vi "Read Sequence Element Configuration.vi"(8 "error in (no error)":errorcluster, 11 "Sequence Element in":refnum<class "Sequence Element.lvclass">) -> (0 "error out":errorcluster, 2 "Configuration":T1 {"Duration" format="%#_6ps"}, 3 "Sequence Element out":refnum<class "Sequence Element.lvclass">)   [LabVIEW 2016, in "Sequence Element.lvclass"]
uses:
  Sequence Element.lvclass
  C:/github/Measure_core/da Base/Template Module.lvclass
  Sequence Element Configuration.ctl
  Template Module/Template Module.lvclass/Template Module.ctl
  Template Module/Read Configuration.vi
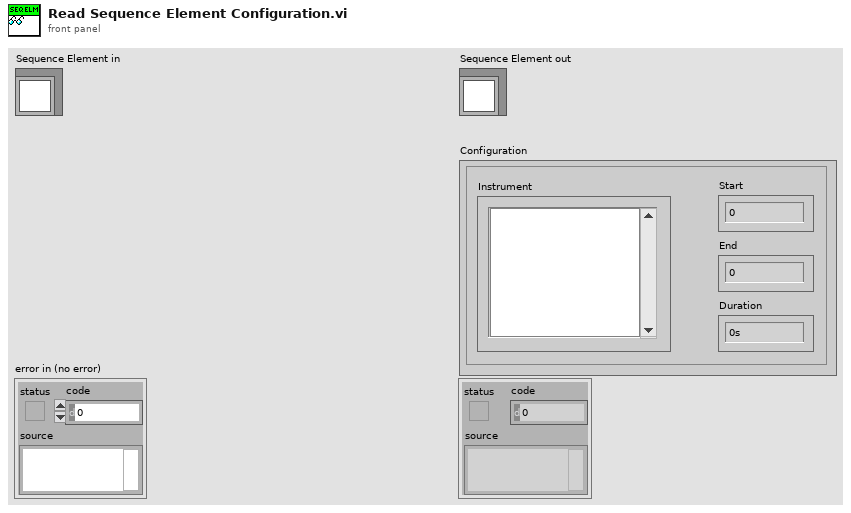
[diagram p1: front panel]
types:
  T1 = typedef "Sequence Element Configuration.ctl" = cluster{"Start":dbl, "End":dbl, "Duration":dbl, "Instrument":i32}
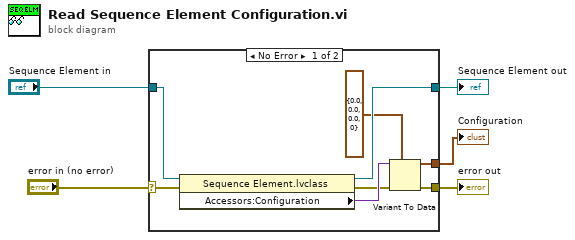
[diagram p0: block diagram]
diagram:
  n1 = case shown="No Error" "error in (no error)" {
    selector: "error in (no error)" -> [w8 w14]
    tunnel: [w6 w14] -> w4
    tunnel: [w12 w15] -> w2
    tunnel: "Sequence Element in" -> [w13 w15]
    tunnel: [w9 _] -> w1
    frame No Error {
      n2 = property class="Sequence Element.lvclass"(reference=w13, error in=w8) -> (reference out=w12:refnum<class "Sequence Element.lvclass">, error out=w7:errorcluster, "Accessors:Configuration"=w11:variant)
      n3 = Variant To Data(error in=w7, type=T1 {"Start"=0.0, "End"=0.0, "Duration"=0.0, "Instrument"=0} ("Configuration"), Variant=w11) -> (data=w9:T1, error out=w6:errorcluster)
    }
    frame Error {
    }
  }
  "error out" <- w4
  "Sequence Element out" <- w2
  "Configuration" <- w1
